vi "Find APU.vi"(8 "error in (no error)":errorcluster, 10 "APU name":string, 11 "EST custom device in":refnum<k24>) -> (0 "error out":errorcluster, 2 "APU Node":refnum<k24>, 3 "EST custom device out":refnum<k24>)   [LabVIEW 2015, in "Engine Simulation Toolkit SysDef API.lvlib"]
uses:
  Engine Simulation Toolkit SysDef API.lvlib
  NationalInstruments.VeriStand.SystemDefinitionAPI
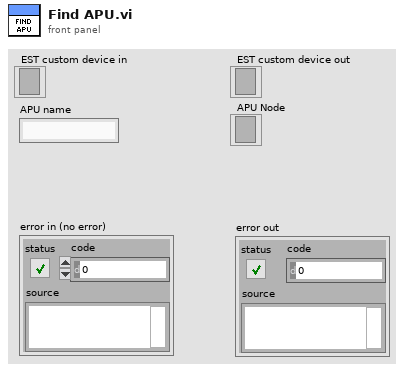
[diagram p1: front panel]
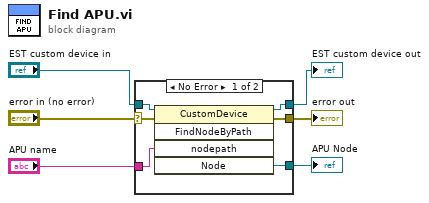
[diagram p0: block diagram]
diagram:
  n1 = case shown="No Error" "error in (no error)" {
    selector: "error in (no error)" -> [w10 w14]
    tunnel: "APU name" -> [w9 _]
    tunnel: "EST custom device in" -> [w7 w13]
    tunnel: [w8 w13] -> w4
    tunnel: [w11 w14] -> w3
    tunnel: [w12 _] -> w1
    frame No Error {
      n2 = invoke class="CustomDevice" method="FindNodeByPath"(reference=w7, error in=w10, "nodepath"=w9) -> (reference out=w8:refnum<k24>, error out=w11:errorcluster, "Node"=w12:refnum<k24>)  [unwired: 2 in, 2 out]
    }
    frame Error {
    }
  }
  "APU Node" <- w1
  "EST custom device out" <- w4
  "error out" <- w3
